vi "RSDC.vi"(0 "Cluster":T1) -> (1 "-Q":bool, 2 "Q":bool)   [LabVIEW 2017]
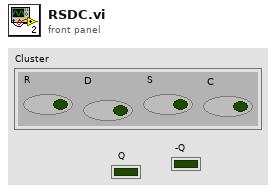
[diagram p1: front panel]
types:
  T1 = cluster{"R":bool, "D ":bool, " S":bool, " C":bool}
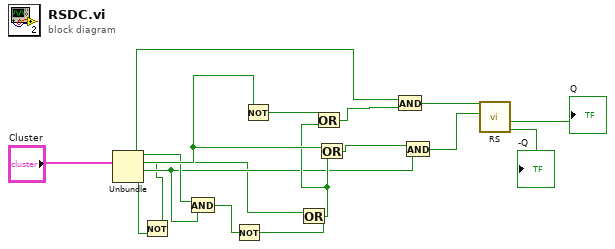
[diagram p0: block diagram]
diagram:
  n1 = Unbundle("Cluster") -> ("R"=w9:bool, "D"=w13:bool, "S"=w7:bool, "C"=w2:bool)
  n2 = Not(x=w2) -> (.not. x?=w1:bool)
  n3 = And(x=w9, y=w7) -> (x .and. y?=w15:bool)
  n4 = Not(x=w15) -> (.not. x?=w14:bool)
  n5 = Not(x=w13) -> (.not. x?=w12:bool)
  n6 = Or(x=w1, y=w14) -> (x .or. y?=w11:bool)
  n7 = Or(x=w12, y=w11) -> (x .or. y?=w10:bool)
  n8 = Or(x=w13, y=w11) -> (x .or. y?=w8:bool)
  n9 = And(x=w9, y=w10) -> (x .and. y?=w6:bool)
  n10 = And(x=w8, y=w7) -> (x .and. y?=w5:bool)
  n11 = call "RS.vi"("S"=w5, "R"=w6) -> ("nQ"=→"-Q":bool, "Q"=→"Q":bool)
